vi "Simple_DAQ_AnalogIO.ProcConstructor.vi"(0 "i ref in":refnum<vi>, 3 "Timeout":i32=10000, 5 "error in":errorcluster caption="Fehler (Eingang, kein Fehler)") -> (14 "i ref out":refnum<vi>, 17 "timed out":bool, 19 "error out":errorcluster caption="Fehler (Ausgang)")   [LabVIEW 2014, in "Simple_DAQ_AnalogIO.lvlib"]
doc: "Contact: Falk Ziegler, eMail: info@lab-coding.de"
uses:
  Simple_DAQ_AnalogIO.lvlib
  CSCore/CSApplicationBaseClasses/PSChannelBase/PSChannelBase.statusType.ctl
  CSlibraries/UtilityLib/UtilityLib.valueStatus.ctl
  CSCore/CSApplicationBaseClasses/PSChannelBase/PSChannelBase.lvlib
  CSlibraries/UtilityLib/UtilityLib.lvlib
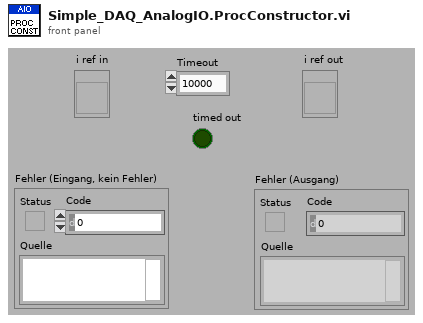
[diagram p1: front panel]
types:
  T1 = typedef "UtilityLib.lvlib/UtilityLib.valueStatus.ctl" = enum16{"no info available", "stand by/off", "on", "warning", "alarm/malfunction", "not implemented", "user action required", "important information", "system default", "control default", "indicator default", "button default"}
  T2 = typedef "PSChannelBase.lvlib/PSChannelBase.statusType.ctl" = i32
  T3 = typedef "Simple_DAQ_AnalogIO.lvlib/Simple_DAQ_AnalogIO.i attribute.ctl" = cluster{"inputs":cluster{"index":i32[], "channel_task":refnum<k21>[], "range":cluster{"min":dbl, "max":dbl}[], "channel_number":i32, "scale_factor":dbl}, "outputs":cluster{"index":i32[], "channel_task":refnum<k21>[], "range":cluster{"min":dbl, "max":dbl}[], "channel_number":i32, "scale_factor":dbl}}
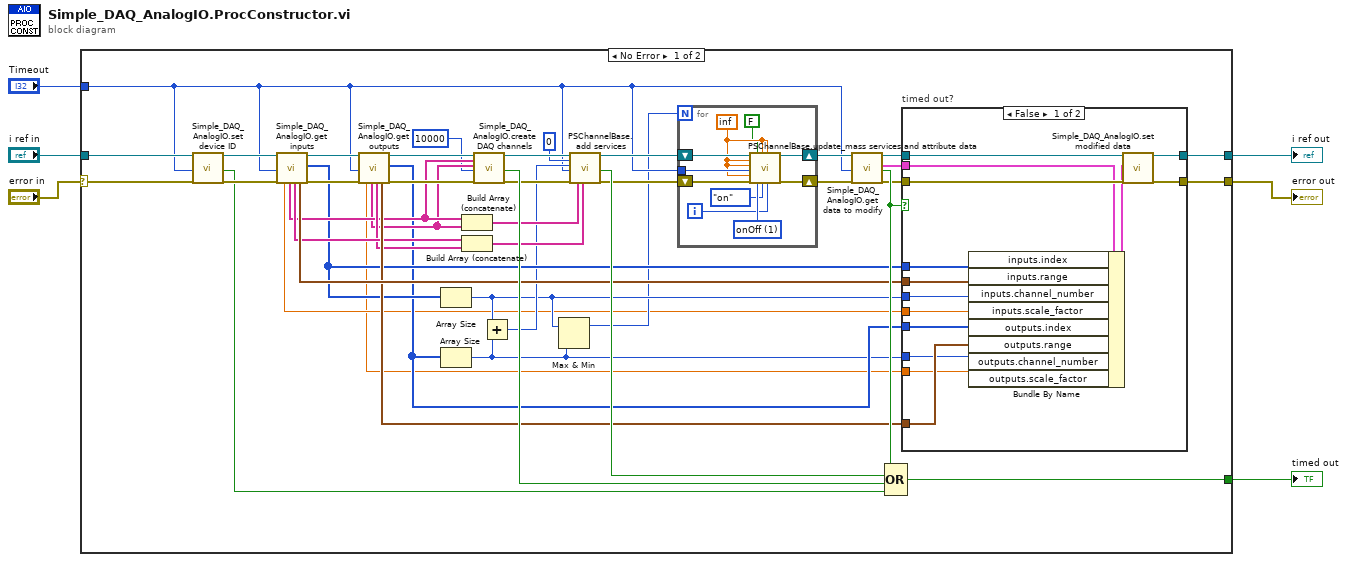
[diagram p0: block diagram]
diagram:
  n1 = case shown="No Error" "error in" {
    selector: "error in" -> [w22 w76]
    tunnel: "i ref in" -> [w25 w77]
    tunnel: [w28 w77] -> w4
    tunnel: [w27 w76] -> w3
    tunnel: "Timeout" -> [w12 _]
    tunnel: [w26 _] -> w1
    frame No Error {
      n2 = call "Simple_DAQ_AnalogIO.set device ID.vi"("i ref in"=w25, "Timeout"=w12, "error in"=w22) -> ("i ref out"=w24:refnum<vi>, "timed out"=w21:bool, "error out"=w23:errorcluster)  [unwired: 14 in]
      n3 = call "Simple_DAQ_AnalogIO.get inputs.vi"("i ref in"=w24, "Timeout"=w12, "error in"=w23) -> ("scale_factor"=w8:dbl, "physical_channels"=w36:string[], "virtual_channels"=w38:string[], "range"=w46:cluster{"min":dbl, "max":dbl}[], "i ref out"=w44:refnum<vi>, "channel_number"=w20:i32[], "error out"=w43:errorcluster)  [unwired: 10 in]
      n4 = call "Simple_DAQ_AnalogIO.get outputs.vi"("i ref in"=w44, "Timeout"=w12, "error in"=w43) -> ("scale_factor"=w7:dbl, "physical_channels"=w35:string[], "virtual_channels"=w37:string[], "range"=w45:cluster{"min":dbl, "max":dbl}[], "i ref out"=w41:refnum<vi>, "channel_index"=w19:i32[], "error out"=w42:errorcluster)  [unwired: 10 in]
      n5 = Array Size(array=w20) -> (size(s)=w11:i32)
      n6 = Array Size(array=w19) -> (size(s)=w10:i32)
      n7 = Build Array (concatenate)(w36, w35) -> (w34:string[])
      n8 = Build Array (concatenate)(w38, w37) -> (w33:string[])
      n9 = call "Simple_DAQ_AnalogIO.create DAQ channels.vi"("i ref in"=w41, "input_channels"=w36, "output_channels"=w35, "Timeout"=10000, "error in"=w42) -> ("i ref out"=w40:refnum<vi>, "timed out"=w47:bool, "error out"=w39:errorcluster)  [unwired: 12 in]
      n10 = Add(x=w11, y=w10) -> (x+y=w13:i32)
      n11 = Max & Min(x=w11, y=w10) -> (max(x,y)=w9:i32)  [unwired: 1 out]
      n12 = call "PSChannelBase.add services.vi"("i ref in"=w40, "defaultChannelIndex"=0, "nofChannels"=w13, "ms timeout (10000)"=w12, "error in (no error)"=w39, "physicalNames"=w34, "logicalNames"=w33) -> ("i ref out"=w17:refnum<vi>, "timed out"=w48:bool, "error out"=w14:errorcluster)  [unwired: 10 in]
      n13 = for {
        N: w9 -> [_]
        shift-right: [w58] -> w16
        shift-left: w17 -> [w59]
        shift-right: [w57] -> w15
        shift-left: w14 -> [w56]
        tunnel: w12 -> [w55]
        i -> [w51]
        w52 = T2 1 items=["onOff"=1, "inRange"=2, "rampingUp"=4, "rampingDown"=8, "tripped"=16, "error"=32] ("status")
        w54 = inf ("rampDownSpeed")
        n14 = call "PSChannelBase.update_mass services and attribute data.vi"("i ref in"=w59, "tripCurrent"=w54, "rampUpSpeed"=w54, "ms timeout (10000)"=w55, "rampDownSpeed"=w54, "error in (no error)"=w56, "onOff"=FALSE, "status"=w52, "voltage"=w54, "valueStatus"=UtilityLib.valueStatus."on", "current"=w54, "channelNumber"=w51) -> ("i ref out"=w58:refnum<vi>, "error out"=w57:errorcluster)  [unwired: 5 in, 1 out]
      }
      n15 = call "Simple_DAQ_AnalogIO.get data to modify.vi"("i ref in"=w16, "ms timeout (10000)"=w12, "error in (no error)"=w15) -> ("i ref out"=w31:refnum<vi>, "i attribute"=w29:T3, "timed out"=w49:bool, "error out"=w30:errorcluster)  [unwired: 13 in]
      n16 = Compound Arithmetic op=OR(w49, w48, w47, w21) -> (w26:bool)
      n17 = case "timed out?" shown="False" w49 {
        tunnel: w31 -> [w73 w75]
        tunnel: w30 -> [w72 w74]
        tunnel: w29 -> [w71 _]
        tunnel: w20 -> [w69 _]
        tunnel: w19 -> [w64 _]
        tunnel: [w68 w75] -> w28
        tunnel: [w67 w74] -> w27
        tunnel: w46 -> [w66 _]
        tunnel: w45 -> [w65 _]
        tunnel: w11 -> [w63 _]
        tunnel: w10 -> [w62 _]
        tunnel: w8 -> [w61 _]
        tunnel: w7 -> [w60 _]
        frame False {
          n18 = Bundle By Name(cluster=w71, "inputs.index"=w69, "inputs.range"=w66, "inputs.channel_number"=w63, "inputs.scale_factor"=w61, "outputs.index"=w64, "outputs.range"=w65, "outputs.channel_number"=w62, "outputs.scale_factor"=w60) -> (w70:T3)
          n19 = call "Simple_DAQ_AnalogIO.set modified data.vi"("i ref in"=w73, "i attribute"=w70, "error in (no error)"=w72) -> ("i ref out"=w68:refnum<vi>, "error out"=w67:errorcluster)  [unwired: 15 in]
        }
        frame True {
        }
      }
    }
    frame Error {
    }
  }
  "error out" <- w3
  "timed out" <- w1
  "i ref out" <- w4
